vi "MegaAwesome_8_28_12aJW.vi"() -> ()   [LabVIEW 2011]
panel:
  in  "Enum":T1(ring)
  in  "Main Tab Control":T2(tab)
  in  "Transfer File":path
  out "Transfer Folder":path
  out "Current State":T3(ring)
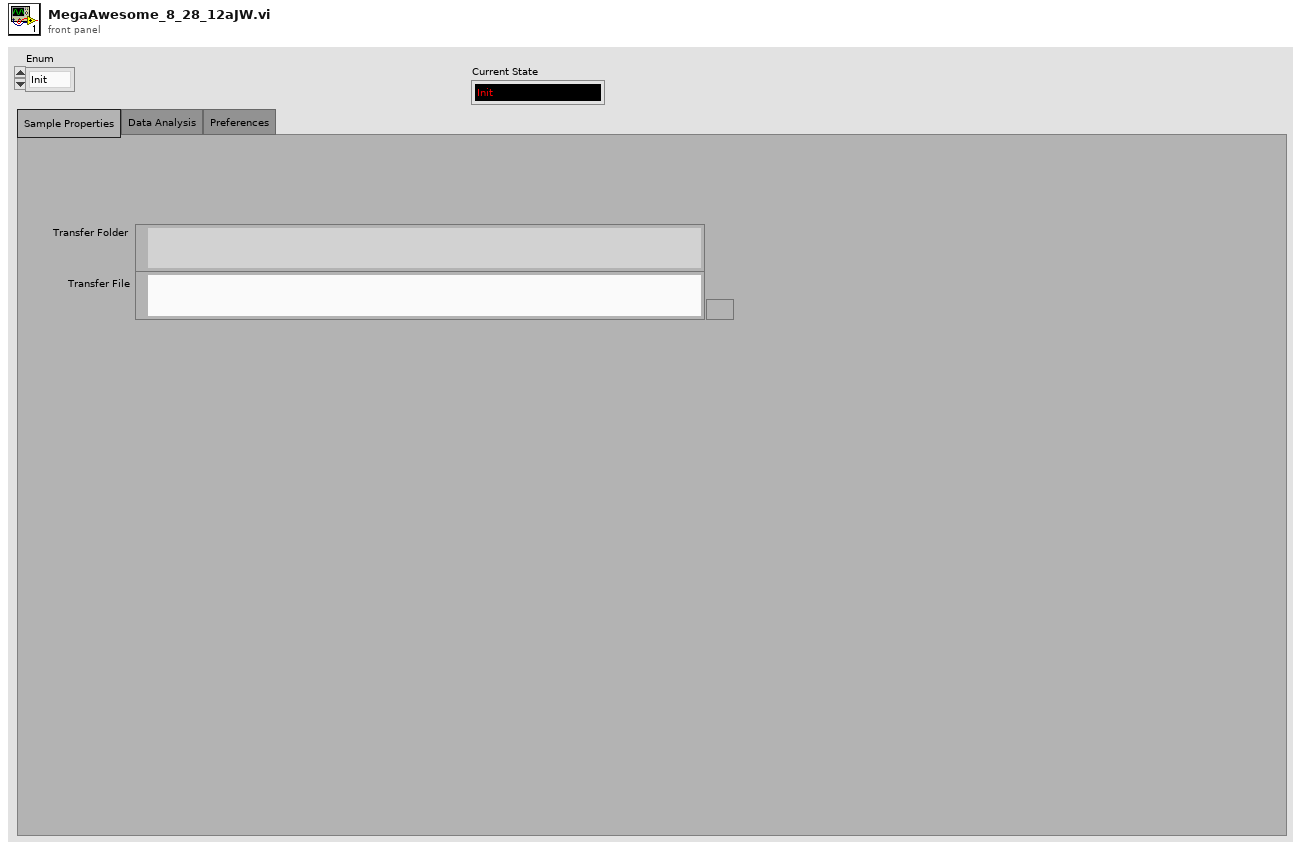
[diagram p1: front panel]
types:
  T1 = enum16{"Init", "File Missing", "No Event", "Exit"}
  T2 = enum32{"Sample Properties", "Data Analysis", "Preferences"}
  T3 = enum16{"Init", "File Missing", "No Event", "Read Data", "Exit"}
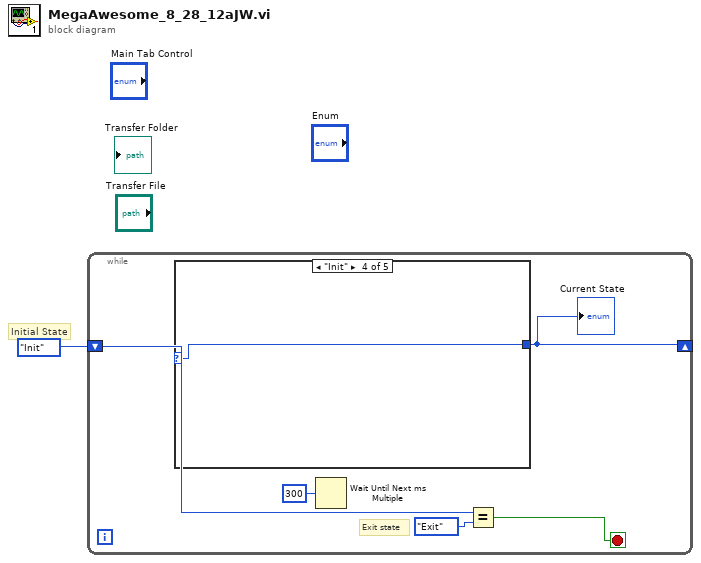
[diagram p0: block diagram]
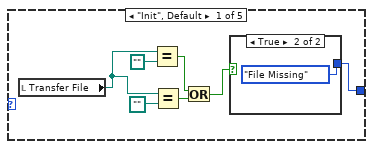
[diagram p2: hidden frame]
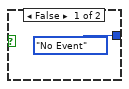
[diagram p3: hidden frame]
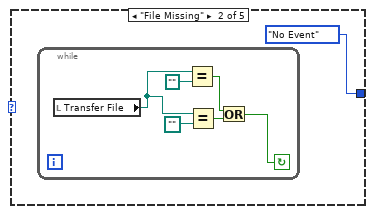
[diagram p4: hidden frame]
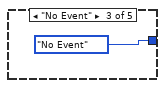
[diagram p5: hidden frame]
diagram:
  # "Initial State"
  n1 = while {
    shift-right: [w3] -> _
    shift-left: T3."Init" -> [w6]
    stop <- w5 stop-if-true
    # "Exit state"
    n2 = case shown="\"Read Data\"" {
      selector: _ -> [_ _ _ w24 w25]
      tunnel: [w7 T1."No Event" T1."No Event" w24 w25] -> w3
      frame "Init", Default {
        n3 = local read "Transfer File"() -> (w9:path)
        n4 = Equal?(x=w9, y=path "") -> (x = y?=w11:bool)
        n5 = Equal?(x=w9, y=path "") -> (x = y?=w12:bool)
        n6 = Or(x=w11, y=w12) -> (x .or. y?=w8:bool)
        n7 = case shown="True" w8 {
          tunnel: [T1."No Event" T1."File Missing"] -> w7
          frame False {
          }
          frame True {
          }
        }
      }
      frame "File Missing" {
        n8 = while {
          stop <- w17 continue-if-true
          n9 = local read "Transfer File"() -> (w18:path)
          n10 = Equal?(x=w18, y=path "") -> (x = y?=w20:bool)
          n11 = Equal?(x=w18, y=path "") -> (x = y?=w21:bool)
          n12 = Or(x=w20, y=w21) -> (x .or. y?=w17:bool)
        }
      }
      frame "No Event" {
      }
      frame "Init" {
      }
      frame "Exit" {
      }
    }
    "Current State" <- w3
    n13 = Wait Until Next ms Multiple(millisecond multiple=u32 300) -> ()  [unwired: 1 out]
    n14 = Equal?(x=w6, y=enum16{"Init", "No Event", "Exit"}."Exit") -> (x = y?=w5:bool)
  }
